vi "RescaleGraphForFourier.vi"(0 "fft reference":refnum<vi>, 2 "fft cluster":T1, 6 "Enum":enum16{"Reciprocal", "Real"}(ring)=enum."Real") -> ()   [LabVIEW 2018, in "myFFT.lvlib"]
uses:
  myFFT.lvlib
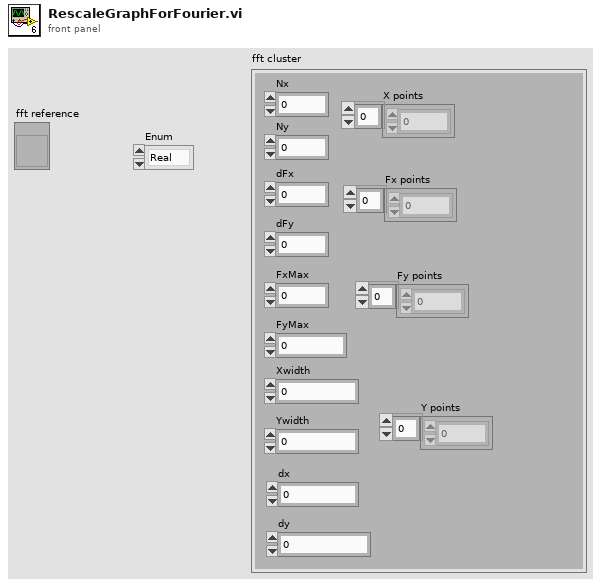
[diagram p1: front panel]
types:
  T1 = cluster{"dFx":dbl, "dFy":dbl, "Nx":i32, "Ny":i32, "FxMax":dbl, "FyMax":dbl, "Xwidth":dbl, "Ywidth":dbl, "dx":dbl, "dy":dbl, "Fx points":dbl[], "X points":dbl[], "Y points":dbl[], "Fy points":dbl[]}
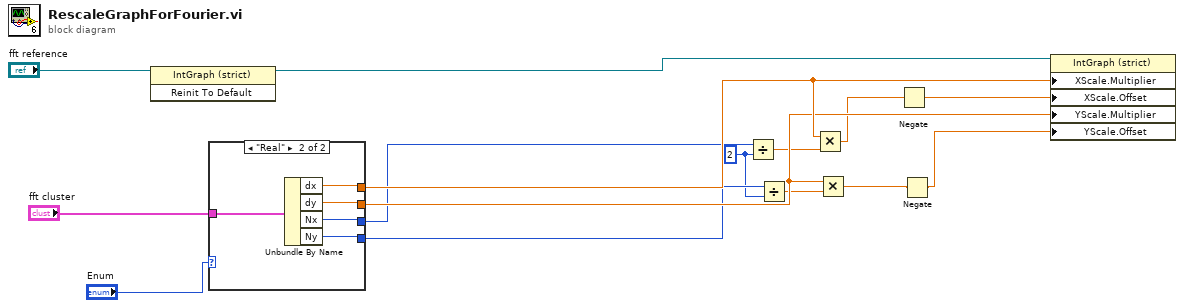
[diagram p0: block diagram]
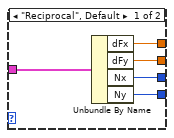
[diagram p2: hidden frame]
diagram:
  w10 = 2 ("y")
  n1 = invoke class="IntGraph (strict)" method="Reinit To Default"(reference="fft reference") -> (reference out=w2:refnum<vi>)  [unwired: 2 in, 2 out]
  n2 = case shown="\"Real\"" "Enum" {
    tunnel: "fft cluster" -> [w20 w25]
    tunnel: [w19 w24] -> w14
    tunnel: [w18 w23] -> w13
    tunnel: [w17 w22] -> w12
    tunnel: [w16 w21] -> w11
    frame "Reciprocal", Default {
      n3 = Unbundle By Name(w20) -> ("dFx"=w19:dbl, "dFy"=w18:dbl, "Nx"=w17:i32, "Ny"=w16:i32)
    }
    frame "Real" {
      n4 = Unbundle By Name(w25) -> ("dx"=w24:dbl, "dy"=w23:dbl, "Nx"=w22:i32, "Ny"=w21:i32)
    }
  }
  n5 = Divide(x=w12, y=w10) -> (x/y=w9:dbl)
  n6 = Divide(x=w11, y=w10) -> (x/y=w8:dbl)
  n7 = Multiply(x=w14, y=w9) -> (x*y=w5:dbl)
  n8 = Multiply(x=w13, y=w8) -> (x*y=w7:dbl)
  n9 = Negate(x=w5) -> (-x=w4:dbl)
  n10 = Negate(x=w7) -> (-x=w6:dbl)
  n11 = property class="IntGraph (strict)"(reference=w2, "XScale.Multiplier"=w14, "XScale.Offset"=w4, "YScale.Multiplier"=w13, "YScale.Offset"=w6) -> ()  [unwired: 1 in, 2 out]
